vi "Interpolate Input[Conflict].vi"(6 "Input Values":dbl[](array[numeric]), 8 "Interpolation Points":cluster{"x":dbl, "y":dbl}[](array[cluster]), 9 "On/Off":bool) -> (0 "Output Values":dbl[](array[numeric]))   [LabVIEW 2018]
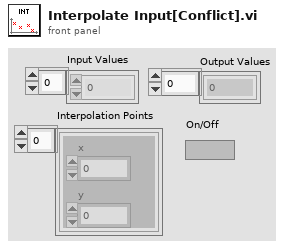
[diagram p1: front panel]
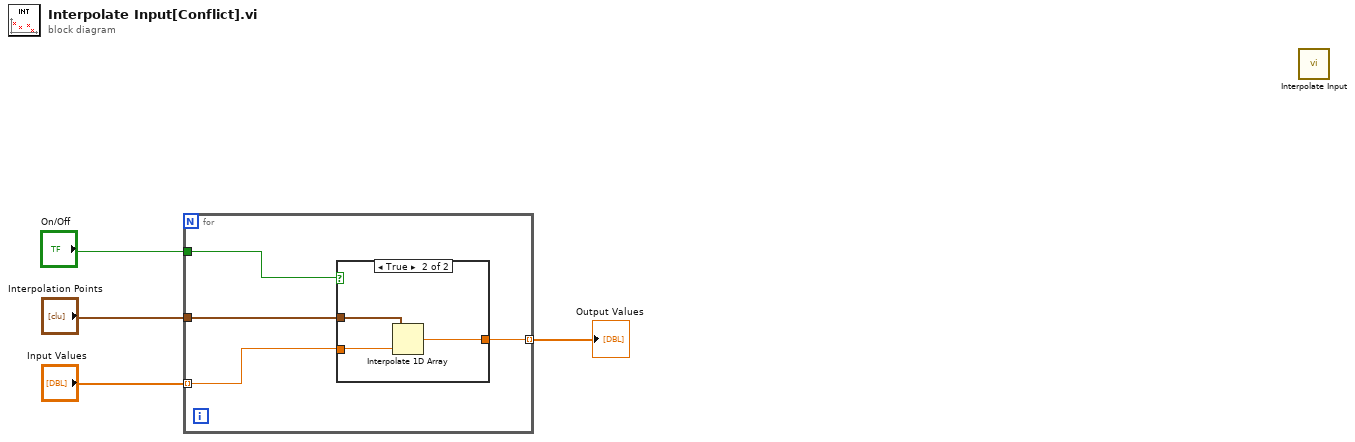
[diagram p0: block diagram]
diagram:
  n1 = for {
    tunnel: "On/Off" -> [w8]
    tunnel: "Interpolation Points" -> [w7]
    tunnel: "Input Values" -> [w6] mode=indexing
    tunnel: [w5] -> w2 mode=indexing
    n2 = case shown="True" w8 {
      tunnel: w7 -> [_ w12]
      tunnel: w6 -> [w9 w11]
      tunnel: [w9 w10] -> w5
      frame False {
      }
      frame True {
        n3 = Interpolate 1D Array(1:w11, 2:w12) -> (0:w10:dbl)
      }
    }
  }
  "Output Values" <- w2
  n4 = call "Interpolate Input.vi"() -> ()  [unwired: 12 in]
